vi "VI Tree.vi"   [LabVIEW 2013, in "Agilent 3446X Series.lvlib"]
doc: "This is the instrument driver for the Agilent 3446X Series. The VI Tree displays all the user-callable VIs of the instrument driver in an organized table."
uses:
  <instrlib>/Agilent 3446X Series/Agilent 3446X Series.lvlib
  <instrlib>/Agilent 3446X Series/Public/Data/Read (Single Point).vi
panel:
  # "(c) 2013-2021 National Instruments.  ALL RIGHTS RESERVED."
  # "SEE DIAGRAM\nFOR VI TREE."
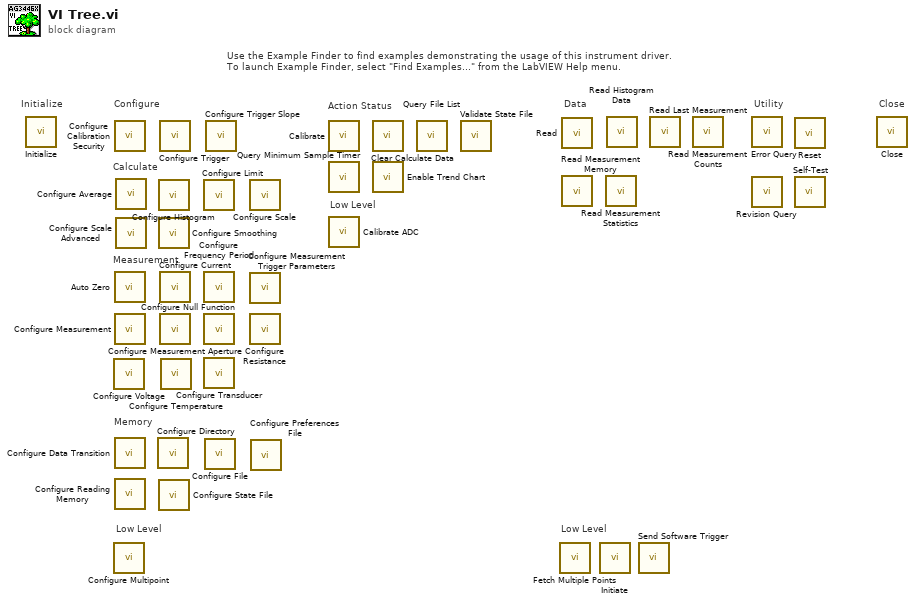
[diagram p0: block diagram]
diagram:
  # "Memory"
  # "Measurement"
  # "Calculate"
  # "Low Level"
  # "Action Status"
  # "Low Level"
  # "Low Level"
  # "Use the Example Finder to find examples demonstrating the usage of this instrument driver.\nTo launch Example Finder, select \"Find Examples...\" from the LabVIEW Help menu."
  # "Configure"
  # "Utility"
  # "Data"
  # "Close"
  # "Initialize"
  n1 = call <instrlib>:"Initialize.vi"() -> ()  [unwired: 10 in, 2 out]
  n2 = call <instrlib>:"Configure Voltage.vi"() -> ()  [unwired: 10 in, 2 out]
  n3 = call <instrlib>:"Configure Multipoint.vi"() -> ()  [unwired: 10 in, 2 out]
  n4 = call <instrlib>:"Configure Calibration Security.vi"() -> ()  [unwired: 10 in, 2 out]
  n5 = call <instrlib>:"Auto Zero.vi"() -> ()  [unwired: 10 in, 2 out]
  n6 = call <instrlib>:"Configure Measurement.vi"() -> ()  [unwired: 10 in, 2 out]
  n7 = call <instrlib>:"Configure Data Transition.vi"() -> ()  [unwired: 10 in, 2 out]
  n8 = call <instrlib>:"Configure Reading Memory.vi"() -> ()  [unwired: 10 in, 2 out]
  n9 = call <instrlib>:"Configure Average.vi"() -> ()  [unwired: 10 in, 2 out]
  n10 = call <instrlib>:"Configure Scale Advanced.vi"() -> ()  [unwired: 10 in, 2 out]
  n11 = call <instrlib>:"Configure Directory.vi"() -> ()  [unwired: 10 in, 2 out]
  n12 = call <instrlib>:"Configure Histogram.vi"() -> ()  [unwired: 10 in, 2 out]
  n13 = call <instrlib>:"Configure Smoothing.vi"() -> ()  [unwired: 10 in, 2 out]
  n14 = call <instrlib>:"Configure State File.vi"() -> ()  [unwired: 10 in, 2 out]
  n15 = call <instrlib>:"Configure Trigger.vi"() -> ()  [unwired: 10 in, 2 out]
  n16 = call <instrlib>:"Configure Current.vi"() -> ()  [unwired: 10 in, 2 out]
  n17 = call <instrlib>:"Configure Measurement Aperture.vi"() -> ()  [unwired: 10 in, 2 out]
  n18 = call <instrlib>:"Configure Temperature.vi"() -> ()  [unwired: 10 in, 2 out]
  n19 = call <instrlib>:"Configure Limit.vi"() -> ()  [unwired: 10 in, 2 out]
  n20 = call <instrlib>:"Configure Frequency Period.vi"() -> ()  [unwired: 10 in, 2 out]
  n21 = call <instrlib>:"Configure Null Function.vi"() -> ()  [unwired: 10 in, 2 out]
  n22 = call <instrlib>:"Configure Transducer.vi"() -> ()  [unwired: 14 in, 2 out]
  n23 = call <instrlib>:"Configure File.vi"() -> ()  [unwired: 10 in, 2 out]
  n24 = call <instrlib>:"Configure Trigger Slope.vi"() -> ()  [unwired: 10 in, 2 out]
  n25 = call <instrlib>:"Configure Scale.vi"() -> ()  [unwired: 10 in, 2 out]
  n26 = call <instrlib>:"Configure Measurement Trigger Parameters.vi"() -> ()  [unwired: 10 in, 2 out]
  n27 = call <instrlib>:"Configure Resistance.vi"() -> ()  [unwired: 10 in, 2 out]
  n28 = call <instrlib>:"Configure Preferences File.vi"() -> ()  [unwired: 10 in, 2 out]
  n29 = call <instrlib>:"Calibrate.vi"() -> ()  [unwired: 9 in, 3 out]
  n30 = call <instrlib>:"Query Minimum Sample Timer.vi"() -> ()  [unwired: 9 in, 3 out]
  n31 = call <instrlib>:"Calibrate ADC.vi"() -> ()  [unwired: 9 in, 3 out]
  n32 = call <instrlib>:"Clear Calculate Data.vi"() -> ()  [unwired: 10 in, 2 out]
  n33 = call <instrlib>:"Enable Trend Chart.vi"() -> ()  [unwired: 10 in, 2 out]
  n34 = call <instrlib>:"Query File List.vi"() -> ()  [unwired: 7 in, 5 out]
  n35 = call <instrlib>:"Validate State File.vi"() -> ()  [unwired: 9 in, 3 out]
  n36 = call <instrlib>:"Fetch Multiple Points.vi"() -> ()  [unwired: 9 in, 3 out]
  n37 = call-poly <instrlib>:"Read.vi"() -> ()  [unwired: 9 in, 3 out]
  n38 = call <instrlib>:"Read Measurement Memory .vi"() -> ()  [unwired: 9 in, 3 out]
  n39 = call <instrlib>:"Initiate.vi"() -> ()  [unwired: 10 in, 2 out]
  n40 = call <instrlib>:"Read Measurement Statistics.vi"() -> ()  [unwired: 8 in, 8 out]
  n41 = call <instrlib>:"Read Histogram Data.vi"() -> ()  [unwired: 9 in, 3 out]
  n42 = call <instrlib>:"Send Software Trigger.vi"() -> ()  [unwired: 10 in, 2 out]
  n43 = call <instrlib>:"Read Last Measurement.vi"() -> ()  [unwired: 9 in, 3 out]
  n44 = call <instrlib>:"Read Measurement Counts.vi"() -> ()  [unwired: 9 in, 3 out]
  n45 = call <instrlib>:"Error Query.vi"() -> ()  [unwired: 8 in, 4 out]
  n46 = call <instrlib>:"Revision Query.vi"() -> ()  [unwired: 8 in, 4 out]
  n47 = call <instrlib>:"Reset.vi"() -> ()  [unwired: 10 in, 2 out]
  n48 = call <instrlib>:"Self-Test.vi"() -> ()  [unwired: 8 in, 4 out]
  n49 = call <instrlib>:"Close.vi"() -> ()  [unwired: 11 in, 1 out]
